vi "GetCfgManagerClassName.vi"(11 "ConfigManager in":refnum<class "ConfigManager.lvclass">) -> (3 "class name":string)   [LabVIEW 2013, in "CfgManager.lvlib" / "ConfigManager.lvclass"]
uses:
  ConfigManager.lvclass
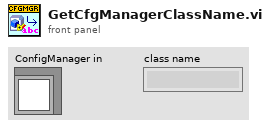
[diagram p1: front panel]
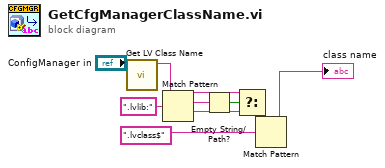
[diagram p0: block diagram]
diagram:
  n1 = call <vilib>:"Get LV Class Name.vi"("object"="ConfigManager in") -> ("class name"=w2:string)  [unwired: 9 in, 1 out]
  n2 = Match Pattern(string=w2, regular expression=".lvlib:") -> (before substring=w6:string, match substring=w4:string, after substring=w7:string)  [unwired: 1 in, 1 out]
  n3 = Empty String/Path?(string/path=w4) -> (empty?=w5:bool)
  n4 = Select(t=w6, s=w5, f=w7) -> (s? t:f=w8:string)
  n5 = Match Pattern(string=w8, regular expression=".lvclass$") -> (before substring=→"class name":string)  [unwired: 1 in, 3 out]
